vi "Final.vi"() -> (1 "輸出分數":dbl)   [LabVIEW 2014]
uses:
  <vilib>/Utility/inputDevices.llb/mouseAcquire.vi
panel:
  out "有沒有按到":bool
  in  "放這裡":string="把碗放這回收"
  in  "開始":string="開始"
  in  "開始倒數":dbl
  in  "倒數計時":dbl
  in  "分數":dbl
  in  "現在吃什麼":dbl
  in  "菜單":cluster{"普通":bool, "巨大":bool, "巨無霸":bool}
  out "axis info":T1
  out "┰难":bool
  in  "這碗麵要吃幾次":dbl
  in  "拉麵被點次數":dbl
  out "button info":T2
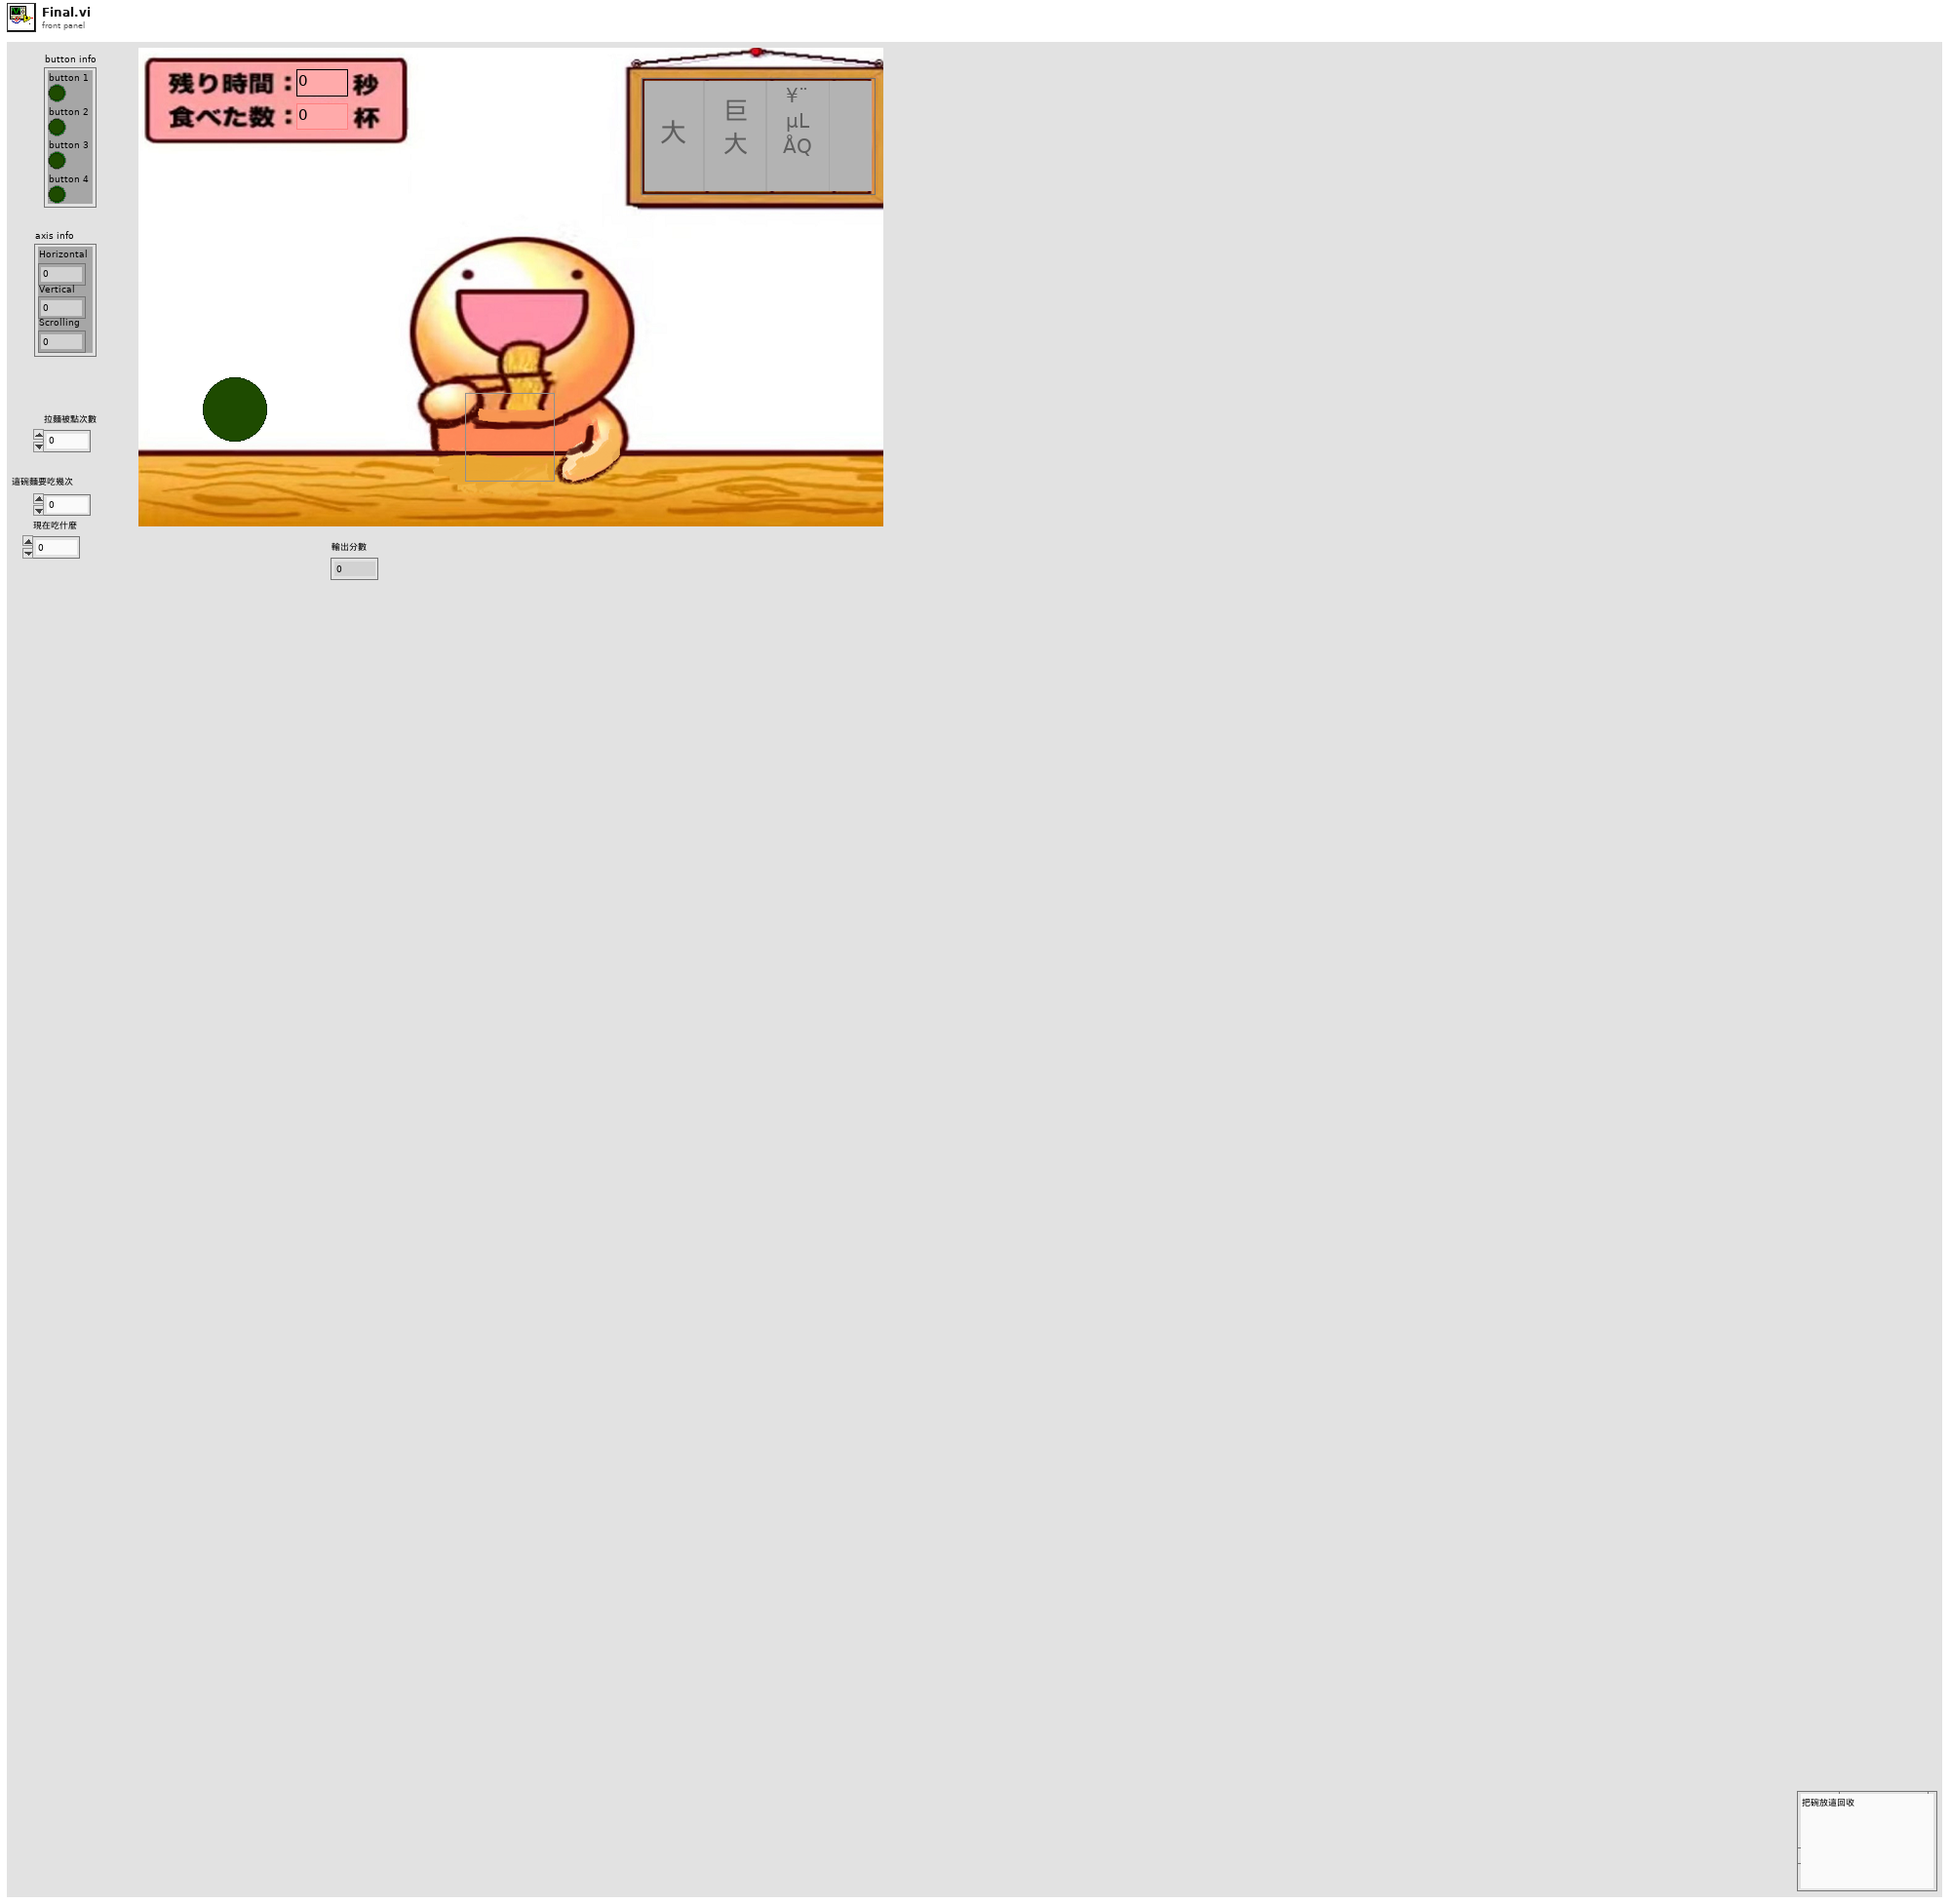
[diagram p1: front panel]
types:
  T1 = cluster{"Horizontal":i32, "Vertical":i32, "Scrolling":i32}
  T2 = cluster{"button 1":bool, "button 2":bool, "button 3":bool, "button 4":bool}
  T3 = enum8{"Enabled", "Disabled", "Disabled and Grayed Out"}
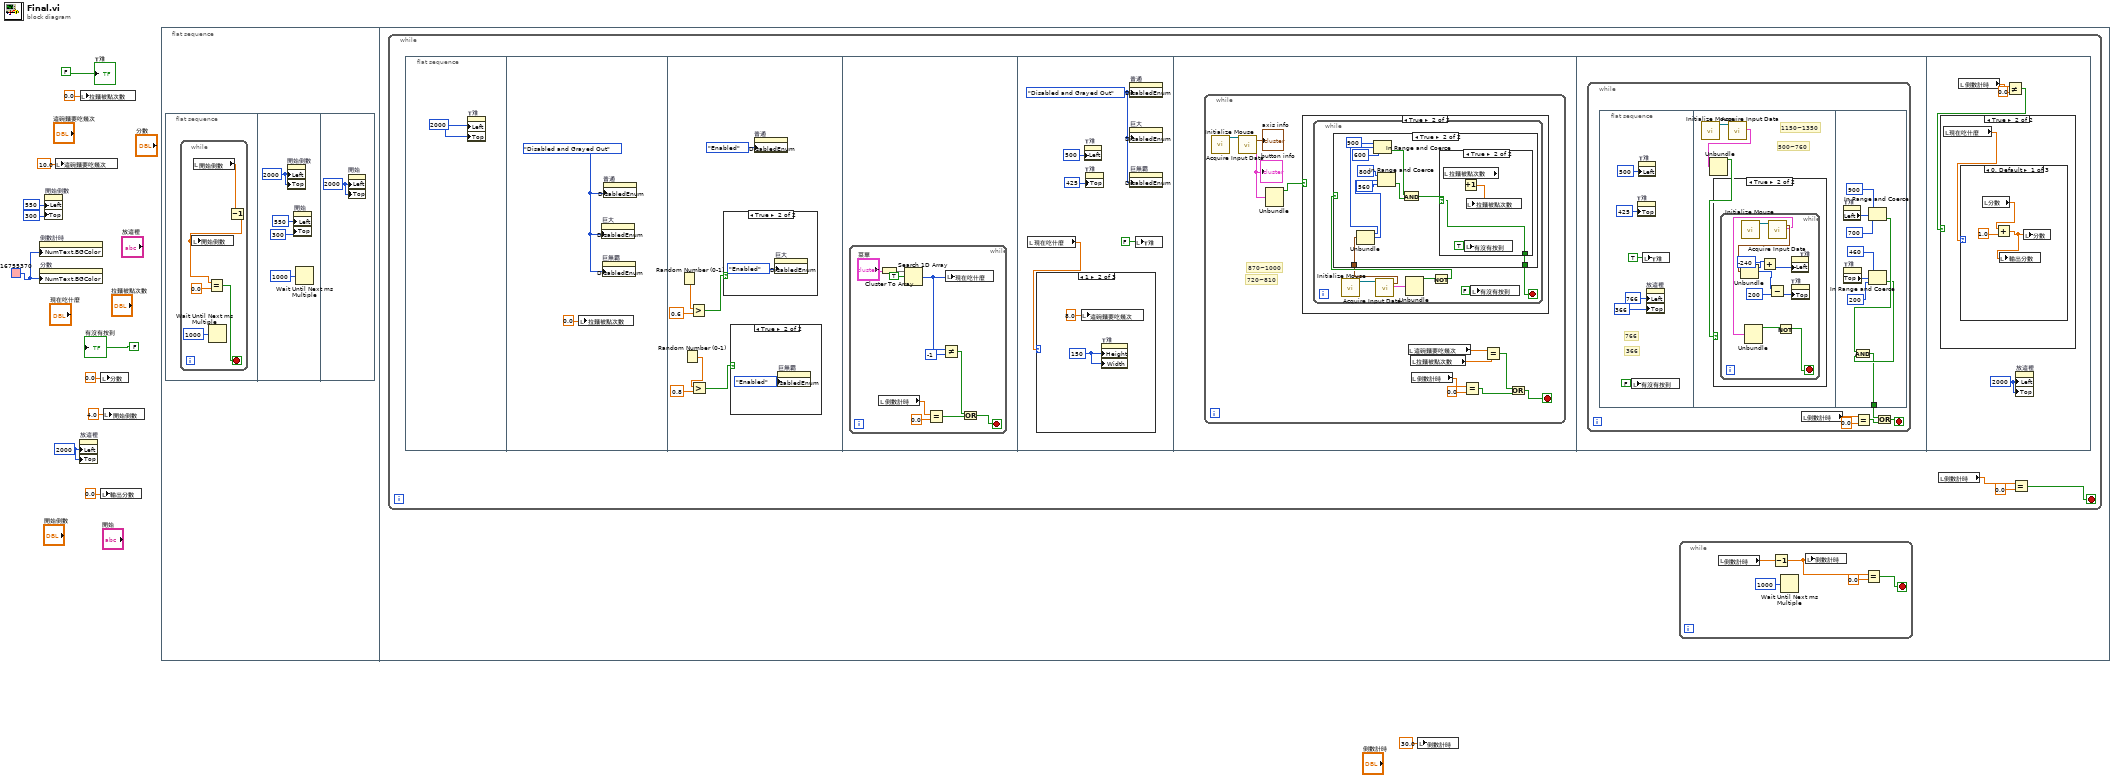
[diagram p0: block diagram]
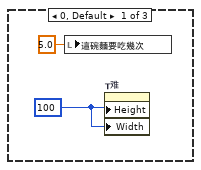
[diagram p4: hidden frame]
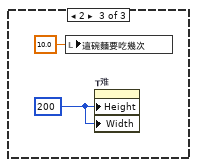
[diagram p5: hidden frame]
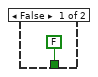
[diagram p7: hidden frame]
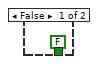
[diagram p8: hidden frame]
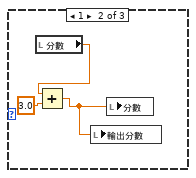
[diagram p11: hidden frame]
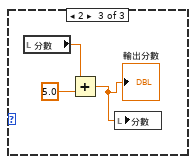
[diagram p12: hidden frame]
diagram:
  w2 = 2000 ("Position:Left")
  w6 = u32 16755370 ("Color Box")
  n1 = property on="倒數計時" class="DigNum (strict)"("NumText.BGColor"=w6) -> ()  [unwired: 2 in, 2 out]
  n2 = property on="分數" class="DigNum (strict)"("NumText.BGColor"=w6) -> ()  [unwired: 2 in, 2 out]
  n3 = property on="開始倒數" class="DigNum (strict)"("Left"=550 ("Position:Left"), "Top"=300 ("Position:Top")) -> ()  [unwired: 2 in, 2 out]
  n4 = local write "這碗麵要吃幾次"(10.0 ("這碗麵還可以吃幾次")) -> ()
  n5 = property on="放這裡" class="Str"("Left"=w2, "Top"=w2) -> ()  [unwired: 2 in, 2 out]
  n6 = local write "拉麵被點次數"(0.0 ("拉麵被點次數")) -> ()
  n7 = local write "輸出分數"(0.0 ("輸出分數")) -> ()
  n8 = local write "分數"(0.0 ("分數")) -> ()
  n9 = local write "開始倒數"(4.0 ("開始倒數")) -> ()
  n10 = flat-sequence {
    frame #0 {
      n11 = flat-sequence {
        frame #0 {
          n12 = while {
            stop <- w13 stop-if-true
            n13 = local read "開始倒數"() -> (w16:dbl)
            n14 = Wait Until Next ms Multiple(millisecond multiple=u32 1000) -> ()  [unwired: 1 out]
            n15 = Decrement(x=w16) -> (x-1=w15:dbl)
            n16 = local write "開始倒數"(w15) -> ()
            n17 = Equal?(x=w15, y=0.0) -> (x = y?=w13:bool)
          }
        }
        frame #1 {
          w21 = 2000 ("Position:Left")
          n18 = property on="開始倒數" class="DigNum (strict)"("Left"=w21, "Top"=w21) -> ()  [unwired: 2 in, 2 out]
          n19 = property on="開始" class="Str"("Left"=550 ("Position:Left"), "Top"=300 ("Position:Top")) -> ()  [unwired: 2 in, 2 out]
          n20 = Wait Until Next ms Multiple(millisecond multiple=u32 1000) -> ()  [unwired: 1 out]
        }
        frame #2 {
          w22 = 2000 ("Position:Left")
          n21 = property on="開始" class="Str"("Left"=w22, "Top"=w22) -> ()  [unwired: 2 in, 2 out]
        }
      }
    }
    frame #1 {
      n22 = while {
        stop <- w28 stop-if-true
        n23 = flat-sequence {
          frame #0 {
            w31 = 2000
            n24 = property on="┰难" class="Bool (strict)"("Left"=w31, "Top"=w31) -> ()  [unwired: 2 in, 2 out]
          }
          frame #1 {
            w33 = T3."Disabled and Grayed Out" ("Disabled")
            n25 = local write "拉麵被點次數"(0.0 ("拉麵被點次數")) -> ()
            n26 = property on="巨大" class="Bool"("DisabledEnum"=w33) -> ()  [unwired: 2 in, 2 out]
            n27 = property on="巨無霸" class="Bool"("DisabledEnum"=w33) -> ()  [unwired: 2 in, 2 out]
            n28 = property on="普通" class="Bool"("DisabledEnum"=w33) -> ()  [unwired: 2 in, 2 out]
          }
          frame #2 {
            n29 = Random Number (0-1)() -> (number: 0 to 1=w39:dbl)
            n30 = Random Number (0-1)() -> (number: 0 to 1=w36:dbl)
            n31 = Greater?(x=w39, y=0.6) -> (0:w37:bool)
            n32 = Greater?(x=w36, y=0.8) -> (0:w34:bool)
            n33 = case shown="True" w37 {
              frame False {
              }
              frame True {
                n34 = property on="巨大" class="Bool"("DisabledEnum"=T3."Enabled" ("Disabled")) -> ()  [unwired: 2 in, 2 out]
              }
            }
            n35 = case shown="True" w34 {
              frame False {
              }
              frame True {
                n36 = property on="巨無霸" class="Bool"("DisabledEnum"=T3."Enabled" ("Disabled")) -> ()  [unwired: 2 in, 2 out]
              }
            }
            n37 = property on="普通" class="Bool"("DisabledEnum"=T3."Enabled" ("Disabled")) -> ()  [unwired: 2 in, 2 out]
          }
          frame #3 {
            n38 = while {
              stop <- w43 stop-if-true
              n39 = local read "倒數計時"() -> (w47:dbl)
              n40 = Cluster To Array(cluster="菜單") -> (array=w51:bool[])
              n41 = Search 1D Array(1D array=w51, element=TRUE) -> (index of element=w49:i32)  [unwired: 1 in]
              n42 = Equal?(x=w47, y=0.0) -> (x = y?=w44:bool)
              n43 = Not Equal?(x=w49, y=-1) -> (x != y?=w45:bool)
              n44 = local write "現在吃什麼"(w49) -> ()
              n45 = Or(x=w45, y=w44) -> (x .or. y?=w43:bool)
            }
          }
          frame #4 {
            w57 = T3."Disabled and Grayed Out" ("Disabled")
            n46 = local read "現在吃什麼"() -> (w56:dbl)
            n47 = case shown="1" w56 {
              frame 0, Default {
                w58 = u32 100 ("Caption.Size:Height")
                n48 = local write "這碗麵要吃幾次"(5.0 ("這碗麵要吃幾次")) -> ()
                n49 = property on="┰难" class="Bool (strict)"("Height"=w58, "Width"=w58) -> ()  [unwired: 2 in, 2 out]
              }
              frame 1 {
                w60 = u32 150 ("Caption.Size:Height")
                n50 = local write "這碗麵要吃幾次"(8.0 ("這碗麵要吃幾次")) -> ()
                n51 = property on="┰难" class="Bool (strict)"("Height"=w60, "Width"=w60) -> ()  [unwired: 2 in, 2 out]
              }
              frame 2 {
                w62 = u32 200 ("Caption.Size:Width")
                n52 = local write "這碗麵要吃幾次"(10.0 ("這碗麵要吃幾次")) -> ()
                n53 = property on="┰难" class="Bool (strict)"("Height"=w62, "Width"=w62) -> ()  [unwired: 2 in, 2 out]
              }
            }
            n54 = property on="┰难" class="Bool (strict)"("Left"=500 ("Position:Left")) -> ()  [unwired: 2 in, 2 out]
            n55 = property on="┰难" class="Bool (strict)"("Top"=425 ("Position:Top")) -> ()  [unwired: 2 in, 2 out]
            n56 = property on="普通" class="Bool"("DisabledEnum"=w57) -> ()  [unwired: 2 in, 2 out]
            n57 = property on="巨大" class="Bool"("DisabledEnum"=w57) -> ()  [unwired: 2 in, 2 out]
            n58 = property on="巨無霸" class="Bool"("DisabledEnum"=w57) -> ()  [unwired: 2 in, 2 out]
            n59 = local write "┰难"(FALSE ("┰难")) -> ()
          }
          frame #5 {
            n60 = while {
              stop <- w64 stop-if-true
              # "720~810"
              # "870~1000"
              n61 = call <vilib>:"Initialize Mouse.vi"() -> ("device ID"=w70:refnum<k1>)  [unwired: 10 in, 1 out]
              n62 = call-poly <vilib>:"Acquire Input Data.vi"("device ID"=w70) -> ("axis info"=→"axis info":T1, "button info"=w74:T2)  [unwired: 15 in, 2 out]
              "button info" <- w74
              n63 = Unbundle(w74) -> ("button 1"=w73:bool)  [unwired: 3 out]
              n64 = case shown="True" w73 {
                frame False {
                }
                frame True {
                  n65 = while {
                    stop <- w77 stop-if-true
                    n66 = call <vilib>:"Initialize Mouse.vi"() -> ("device ID"=w81:refnum<k1>)  [unwired: 10 in, 1 out]
                    n67 = call-poly <vilib>:"Acquire Input Data.vi"("device ID"=w81) -> ("axis info"=w76:T1, "button info"=w80:T2)  [unwired: 15 in, 2 out]
                    n68 = Unbundle(w80) -> ("button 1"=w79:bool)  [unwired: 3 out]
                    n69 = Not(x=w79) -> (.not. x?=w78:bool)
                    n70 = case shown="True" w78 {
                      tunnel: [FALSE w87] -> w77
                      tunnel: w76 -> [_ w86]
                      frame False {
                      }
                      frame True {
                        n71 = Unbundle(w86) -> ("Horizontal"=w85:i32, "Vertical"=w83:i32)  [unwired: 1 out]
                        n72 = In Range and Coerce(upper limit=900, x=w85, lower limit=600) -> (In Range?=w92:bool)  [unwired: 1 out]
                        n73 = In Range and Coerce(upper limit=800 ("Vertical"), x=w83, lower limit=560) -> (In Range?=w89:bool)  [unwired: 1 out]
                        n74 = And(x=w92, y=w89) -> (x .and. y?=w88:bool)
                        n75 = case shown="True" w88 {
                          selector: w88 -> [_ w96]
                          tunnel: [FALSE w96] -> w87
                          frame False {
                          }
                          frame True {
                            n76 = local read "拉麵被點次數"() -> (w98:dbl)
                            n77 = Increment(x=w98) -> (x+1=w97:dbl)
                            n78 = local write "有沒有按到"(TRUE ("Boolean")) -> ()
                            n79 = local write "拉麵被點次數"(w97) -> ()
                          }
                        }
                      }
                    }
                    n80 = local write "有沒有按到"(FALSE ("Boolean")) -> ()
                  }
                }
              }
              n81 = local read "這碗麵要吃幾次"() -> (w72:dbl)
              n82 = local read "拉麵被點次數"() -> (w71:dbl)
              n83 = local read "倒數計時"() -> (w68:dbl)
              n84 = Equal?(x=w68, y=0.0) -> (x = y?=w66:bool)
              n85 = Equal?(x=w72, y=w71) -> (x = y?=w65:bool)
              n86 = Or(x=w65, y=w66) -> (x .or. y?=w64:bool)
            }
          }
          frame #6 {
            n87 = while {
              stop <- w99 stop-if-true
              n88 = flat-sequence {
                tunnel: [w124] -> w103
                frame #0 {
                  # "366"
                  # "766"
                  n89 = local write "有沒有按到"(FALSE ("Boolean")) -> ()
                  n90 = property on="┰难" class="Bool (strict)"("Top"=425 ("Position:Top")) -> ()  [unwired: 2 in, 2 out]
                  n91 = property on="┰难" class="Bool (strict)"("Left"=500 ("Position:Left")) -> ()  [unwired: 2 in, 2 out]
                  n92 = local write "┰难"(TRUE ("┰难")) -> ()
                  n93 = property on="放這裡" class="Str"("Left"=766 ("Position:Left"), "Top"=366 ("Position:Top")) -> ()  [unwired: 2 in, 2 out]
                }
                frame #1 {
                  # "500~760"
                  # "1150~1350"
                  n94 = call <vilib>:"Initialize Mouse.vi"() -> ("device ID"=w112:refnum<k1>)  [unwired: 10 in, 1 out]
                  n95 = call-poly <vilib>:"Acquire Input Data.vi"("device ID"=w112) -> ("button info"=w111:T2)  [unwired: 15 in, 3 out]
                  n96 = Unbundle(w111) -> ("button 1"=w110:bool)  [unwired: 3 out]
                  n97 = case shown="True" w110 {
                    frame False {
                    }
                    frame True {
                      n98 = while {
                        stop <- w119 stop-if-true
                        n99 = call <vilib>:"Initialize Mouse.vi"() -> ("device ID"=w123:refnum<k1>)  [unwired: 10 in, 1 out]
                        n100 = call-poly <vilib>:"Acquire Input Data.vi"("device ID"=w123) -> ("axis info"=w122:T1, "button info"=w121:T2)  [unwired: 15 in, 2 out]
                        n101 = Unbundle(w122) -> ("Horizontal"=w117:i32, "Vertical"=w114:i32)  [unwired: 1 out]
                        n102 = Unbundle(w121) -> ("button 1"=w120:bool)  [unwired: 3 out]
                        n103 = Add(x=w117, y=-240) -> (x+y=w118:i32)
                        n104 = Subtract(x=w114, y=200) -> (x-y=w115:i32)
                        n105 = Not(x=w120) -> (.not. x?=w119:bool)
                        n106 = property on="┰难" class="Bool (strict)"("Top"=w115) -> ()  [unwired: 2 in, 2 out]
                        n107 = property on="┰难" class="Bool (strict)"("Left"=w118) -> ()  [unwired: 2 in, 2 out]
                      }
                    }
                  }
                }
                frame #2 {
                  n108 = property on="┰难" class="Bool (strict)"() -> ("Left"=w132:i32)  [unwired: 2 in, 2 out]
                  n109 = property on="┰难" class="Bool (strict)"() -> ("Top"=w129:i32)  [unwired: 2 in, 2 out]
                  n110 = In Range and Coerce(upper limit=900, x=w132, lower limit=700) -> (In Range?=w126:bool)  [unwired: 1 out]
                  n111 = In Range and Coerce(upper limit=460, x=w129, lower limit=200) -> (In Range?=w125:bool)  [unwired: 1 out]
                  n112 = And(x=w126, y=w125) -> (x .and. y?=w124:bool)
                }
              }
              n113 = local read "倒數計時"() -> (w101:dbl)
              n114 = Equal?(x=w101, y=0.0) -> (x = y?=w102:bool)
              n115 = Or(x=w103, y=w102) -> (x .or. y?=w99:bool)
            }
          }
          frame #7 {
            w133 = 2000 ("Position:Left")
            n116 = local read "倒數計時"() -> (w136:dbl)
            n117 = Not Equal?(x=w136, y=0.0) -> (x != y?=w134:bool)
            n118 = case shown="True" w134 {
              frame False {
              }
              frame True {
                n119 = local read "現在吃什麼"() -> (w137:dbl)
                n120 = case shown="0, Default" w137 {
                  frame 0, Default {
                    n121 = local read "分數"() -> (w140:dbl)
                    n122 = Add(x=w140, y=1.0) -> (x+y=w138:dbl)
                    n123 = local write "輸出分數"(w138) -> ()
                    n124 = local write "分數"(w138) -> ()
                  }
                  frame 1 {
                    n125 = local read "分數"() -> (w143:dbl)
                    n126 = Add(x=w143, y=3.0) -> (x+y=w141:dbl)
                    n127 = local write "輸出分數"(w141) -> ()
                    n128 = local write "分數"(w141) -> ()
                  }
                  frame 2 {
                    n129 = local read "分數"() -> (w146:dbl)
                    n130 = Add(x=w146, y=5.0) -> (x+y=w144:dbl)
                    "輸出分數" <- w144
                    n131 = local write "分數"(w144) -> ()
                  }
                }
              }
            }
            n132 = property on="放這裡" class="Str"("Left"=w133, "Top"=w133) -> ()  [unwired: 2 in, 2 out]
          }
        }
        n133 = local read "倒數計時"() -> (w30:dbl)
        n134 = Equal?(x=w30, y=0.0) -> (x = y?=w28:bool)
      }
      n135 = while {
        stop <- w24 stop-if-true
        n136 = local read "倒數計時"() -> (w26:dbl)
        n137 = Decrement(x=w26) -> (x-1=w23:dbl)
        n138 = Wait Until Next ms Multiple(millisecond multiple=u32 1000) -> ()  [unwired: 1 out]
        n139 = local write "倒數計時"(w23) -> ()
        n140 = Equal?(x=w23, y=0.0) -> (x = y?=w24:bool)
      }
    }
  }
  n141 = local write "倒數計時"(30.0 ("倒數計時")) -> ()
  "┰难" <- FALSE ("┰难")
  "有沒有按到" <- FALSE ("Boolean")
